vi "SpectroMeterInit.vi"(0 "LightField Automation in":refnum<class "LightField Automation.lvclass">, 1 "error in":errorcluster) -> (2 "LightField Automation out":refnum<class "LightField Automation.lvclass">, 3 "error out 2":errorcluster, 4 "Queue Reference":refnum<queue>)   [LabVIEW 2018]
uses:
  C:/ProgramData/Documents/Princeton Instruments/LightField/Add-in and Automation SDK/Samples/LabVIEW Automation/lightfield-automation-labview/LightField Automation.lvclass
panel:
  in  "error in (no error)":errorcluster
  out "current grating center":dbl
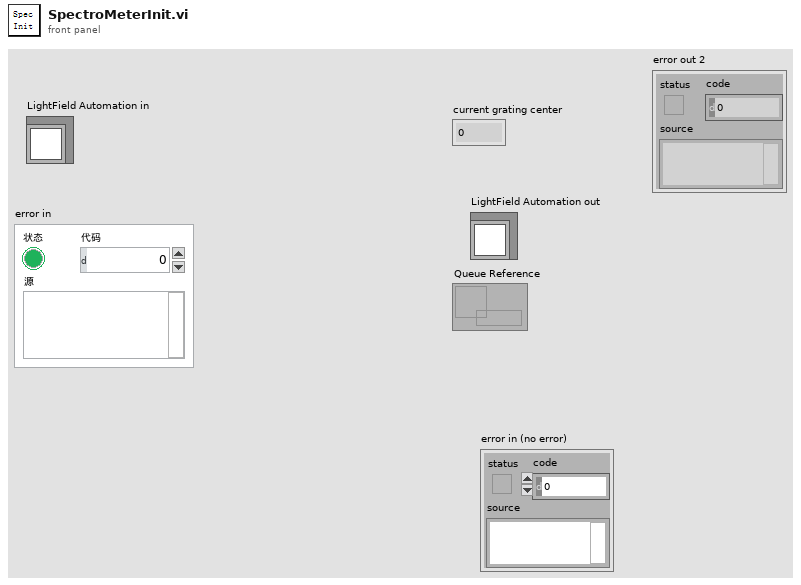
[diagram p1: front panel]
types:
  T1 = typedef "IMAQ Image.ctl" = refnum<image>
  T2 = cluster{"示波器":cluster{"Channel (0:Channel 1)":enum16{"Channel 1", "Channel 2", "Channel 3", "Channel 4"}, "电压范围":dbl, "触发电压":dbl, "时间范围":dbl, " 示波器VISA":refnum<visa-resource-name>, "时间范围 标签":u64, "电压范围 标签":u64, "触发电压 标签":u64, "输入阻抗/Ω":u64}, "光谱仪":cluster{"SpecDataReference":refnum<queue>, "grating center":dbl, "Exposure Time (s)":dbl, "是否进行详细设置":bool, " 开始通信检查":bool, "通信成功？":bool, "波长":dbl}, " 近场相机":cluster{"曝光时间/100us":dbl, "模拟增益":i32, "控制套接字":i32, "IP 地址":string, " 采集套接字":i32, "  版本号":i32, "ImageData":T1, "  增益最大":i32, "  增益最小":i32, " 曝光最大":i32, " 曝光最小":i32, " 帧速":i32, " 同步切换":i32, "  曝光缩放":i32}, " 偏振仪":cluster{"电压范围":u64, "触发电压":u64, "时间范围":u64, "波长范围":enum16{"可见光 400-700nm", "近红外 700-1100nm"}, "可见光偏振测量仪VISA":refnum<visa-resource-name>, "近红外偏振测量仪VISA":refnum<visa-resource-name>}, " 功率计":cluster{"通道":enum16{"Channel 1", "Channel 2"}, "工作波长":u32, "单位":u64, "时间范围":u64, "IP地址":string, "端口":u32}, "能量计":cluster{"通道":enum16{"Channel 1", "Channel 2"}, "工作波长":u32, "单位":u64, "时间范围":u64, "IP地址":string, "端口":u32, "能量计量程":enum16{"200uJ", "20uJ", "2uJ", "200nJ"}}, "电机":cluster{"Channel (0:Channel 1)":enum16{"Channel 1", "Channel 2", "Channel 3", "Channel 4"}, "电压范围":u64, "触发电压":u64, "时间范围":u64}, " 远场相机":cluster{"曝光时间":i32, "模拟增益":i32, "控制套接字":i32, "IP 地址":string, " 采集套接字":i32, "  版本号":i32, "ImageData":T1, "  增益最大":i32, "  增益最小":i32, " 曝光最大":i32, " 曝光最小":i32, " 帧速":i32, " 同步切换":i32, "  曝光缩放":i32, "ImageData B":T1}}
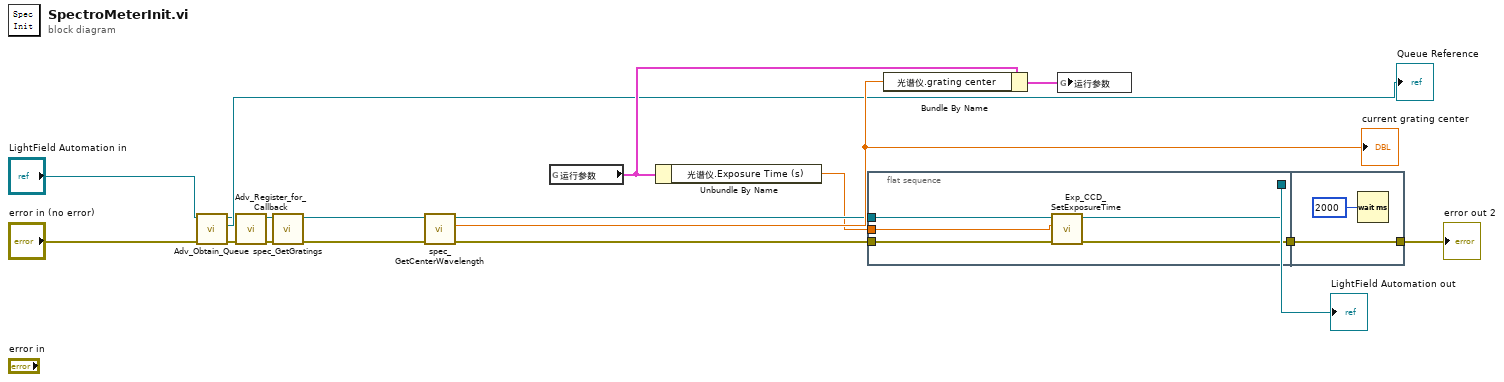
[diagram p0: block diagram]
diagram:
  n1 = call "Adv_Obtain_Queue.vi"("error in (no error)"="error in (no error)", "LightField Automation in"="LightField Automation in") -> ("error out"=w5:errorcluster, "Queue Reference"=→"Queue Reference":refnum<queue>, "LightField Automation out"=w6:refnum<class "LightField Automation.lvclass">)  [unwired: 7 in]
  n2 = call "Adv_Register_for_Callback.vi"("error in (no error)"=w5, "LightField Automation in"=w6) -> ("error out"=w3:errorcluster, "LightField Automation out"=w4:refnum<class "LightField Automation.lvclass">)  [unwired: 8 in]
  n3 = call "spec_GetGratings.vi"("error in (no error)"=w3, "LightField Automation in"=w4) -> ("error out"=w17:errorcluster, "LightField Automation out"=w18:refnum<class "LightField Automation.lvclass">)  [unwired: 6 in, 2 out]
  n4 = call "spec_GetCenterWavelength.vi"("error in (no error)"=w17, "LightField Automation in"=w18) -> ("error out"=w12:errorcluster, "Center Wavelenght"=w15:dbl, "LightField Automation out"=w13:refnum<class "LightField Automation.lvclass">)  [unwired: 7 in]
  "current grating center" <- w15
  n5 = global read "参数.vi" "运行参数"() -> (w16:T2)
  n6 = Unbundle By Name(w16) -> ("光谱仪.Exposure Time (s)"=w9:dbl)
  n7 = flat-sequence {
    tunnel: w13 -> [w23]
    tunnel: w12 -> [w22]
    tunnel: [w21] -> w11
    tunnel: w9 -> [w19]
    tunnel: [w20] -> w8
    tunnel: [w25] -> w10
    tunnel: w8 -> [w25]
    frame #0 {
      n8 = call "Exp_CCD_SetExposureTime.vi"("error in (no error)"=w22, "Exposure Time (s)"=w19, "LightField Automation in"=w23) -> ("error out"=w20:errorcluster, "LightField Automation out"=w21:refnum<class "LightField Automation.lvclass">)  [unwired: 7 in]
    }
    frame #1 {
      n9 = Wait (ms)(milliseconds to wait=u32 2000 ("等待时间（毫秒）")) -> ()  [unwired: 1 out]
    }
  }
  n10 = Bundle By Name(cluster=w16, "光谱仪.grating center"=w15) -> (w14:T2)
  n11 = global write "参数.vi" "运行参数"(w14) -> ()
  "LightField Automation out" <- w11
  "error out 2" <- w10
